vi "RegisterLicense.vi"(7 "key":string, 8 "licensee":string, 10 "error in":errorcluster) -> (3 "error out":errorcluster)   [LabVIEW 2023, in "UnderAutomation.UniversalRobots.lvlib"]
uses:
  UnderAutomation.UniversalRobots.lvlib
  C:/Users/fg/Documents/UniversalRobots.vi/UnderAutomation.UniversalRobots/lib/UnderAutomation.UniversalRobots.dll
  lib/UnderAutomation.UniversalRobots.dll
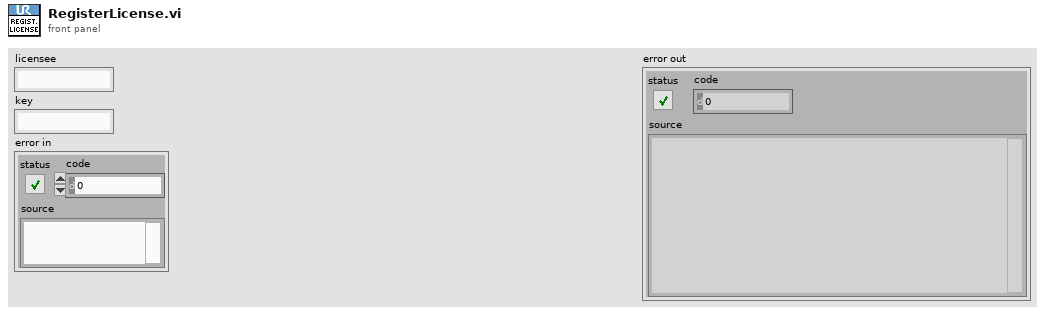
[diagram p1: front panel]
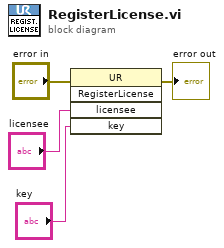
[diagram p0: block diagram]
diagram:
  n1 = invoke class="UR" method="RegisterLicense"(error in="error in", "licensee"="licensee", "key"="key") -> (error out=→"error out":errorcluster)  [unwired: 2 in, 4 out]
